vi "svx_ZScale.Multiplier Write.vi"(4 "error in (no error)":errorcluster, 5 "Value":dbl, 6 "Container State":T3, 7 "Display State In":T1={"X Scale Width %"=50.0, "Y Scale Height %"=50.0, "X-Axis Range"={"Minimum"=0.0, "Maximum"=10.0}, "Y-Axis Range"={"Minimum"=0.0, "Maximum"=10.0}, "Z-Axis Range"={"Minimum"=0.0, "Maximum"=10.0}, "Plot Color"=61212, "Frame Color"=16252785, "Background Color"=16777222, "Initial AutoScale Y"=TRUE, "AutoScale X"=2, "AutoScale Y"=2, "AutoScale Z"=2, "Plot Transparency"=FALSE, "X-Axis Name"="Frequency", "Y-Axis Name"="Amplitude", "Z-Axis Name"="", "X-Axis Scaling Factor"={"Offset"=0.0, "Multiplier"=1.0}, "Y-Axis Scaling Factor"={"Offset"=0.0, "Multiplier"=1.0}, "Z-Axis Scaling Factor"={"Offset"=0.0, "Multiplier"=1.0}, "X-Scale Visible"=TRUE, "Y-Scale Visible"=TRUE, "Z-Scale Visible"=TRUE, "X-Scale Label Visible"=TRUE, "Y-Scale Label Visible"=TRUE, "Z-Scale Label Visible"=TRUE, "X-Axis Range Scaled"={"Minimum"=0.0, "Maximum"=10.0}, "Y-Axis Range Scaled"={"Minimum"=0.0, "Maximum"=10.0}, "Z-Axis Range Scaled"={"Minimum"=0.0, "Maximum"=10.0}, "Rev Z Order"=FALSE, "X-Scale Format Str"="%#.4g", "Y-Scale Format Str"="%#.4g", "Z-Scale Format Str"="%#.4g", "Decor color"=12369084, "Scale Range Change"=refnum, "out of state queue"=refnum, "property nodes"=refnum, "Lines"=[], "Line Properties"={"Line Color"=61212, "Line Width"=61212, "Line Style"=enum."Dash", "DisplayLines"=FALSE}} {"Line Properties"."Line Width" min=1}) -> (0 "error out":errorcluster, 3 "Display State Out":T1={"X Scale Width %"=50.0, "Y Scale Height %"=50.0, "X-Axis Range"={"Minimum"=0.0, "Maximum"=10.0}, "Y-Axis Range"={"Minimum"=0.0, "Maximum"=10.0}, "Z-Axis Range"={"Minimum"=0.0, "Maximum"=10.0}, "Plot Color"=61212, "Frame Color"=16252785, "Background Color"=16777222, "Initial AutoScale Y"=TRUE, "AutoScale X"=2, "AutoScale Y"=2, "AutoScale Z"=2, "Plot Transparency"=FALSE, "X-Axis Name"="Frequency", "Y-Axis Name"="Amplitude", "Z-Axis Name"="", "X-Axis Scaling Factor"={"Offset"=0.0, "Multiplier"=1.0}, "Y-Axis Scaling Factor"={"Offset"=0.0, "Multiplier"=1.0}, "Z-Axis Scaling Factor"={"Offset"=0.0, "Multiplier"=1.0}, "X-Scale Visible"=TRUE, "Y-Scale Visible"=TRUE, "Z-Scale Visible"=TRUE, "X-Scale Label Visible"=TRUE, "Y-Scale Label Visible"=TRUE, "Z-Scale Label Visible"=TRUE, "X-Axis Range Scaled"={"Minimum"=0.0, "Maximum"=10.0}, "Y-Axis Range Scaled"={"Minimum"=0.0, "Maximum"=10.0}, "Z-Axis Range Scaled"={"Minimum"=0.0, "Maximum"=10.0}, "Rev Z Order"=FALSE, "X-Scale Format Str"="%#.4g", "Y-Scale Format Str"="%#.4g", "Z-Scale Format Str"="%#.4g", "Decor color"=12369084, "Scale Range Change"=refnum, "out of state queue"=refnum, "property nodes"=refnum, "Lines"=[], "Line Properties"={"Line Color"=61212, "Line Width"=61212, "Line Style"=enum."Dash", "DisplayLines"=FALSE}} {"Line Properties"."Line Width" min=1})   [LabVIEW 2017, in "SVX Waterfall Graph.xctl"]
uses:
  <vilib>/addons/_XControls/Waterfall Graph/SVX Waterfall Graph.xctl
  <vilib>/_xctls/Container State.ctl
  <vilib>/addons/_XControls/Waterfall Graph/subVIs/svx_Waterfall State.ctl
  <vilib>/addons/_NISVFA/_Shared subVIs/Controls/svc_Cluster of Array of Cluster of XYZ.ctl
  <vilib>/_xctls/XControlSupport.lvlib
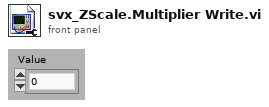
[diagram p1: front panel]
types:
  T1 = typedef "SVX Waterfall Graph.xctl/svx_Waterfall State.ctl" = cluster{"X Scale Width %":dbl, "Y Scale Height %":dbl, "X-Axis Range":cluster{"Minimum":dbl, "Maximum":dbl}, "Y-Axis Range":cluster{"Minimum":dbl, "Maximum":dbl}, "Z-Axis Range":cluster{"Minimum":dbl, "Maximum":dbl}, "Plot Color":u32, "Frame Color":u32, "Background Color":u32, "Initial AutoScale Y":bool, "AutoScale X":u8, "AutoScale Y":u8, "AutoScale Z":u8, "Plot Transparency":bool, "X-Axis Name":string, "Y-Axis Name":string, "Z-Axis Name":string, "X-Axis Scaling Factor":cluster{"Offset":dbl, "Multiplier":dbl}, "Y-Axis Scaling Factor":cluster{"Offset":dbl, "Multiplier":dbl}, "Z-Axis Scaling Factor":cluster{"Offset":dbl, "Multiplier":dbl}, "X-Scale Visible":bool, "Y-Scale Visible":bool, "Z-Scale Visible":bool, "X-Scale Label Visible":bool, "Y-Scale Label Visible":bool, "Z-Scale Label Visible":bool, "X-Axis Range Scaled":cluster{"Minimum":dbl, "Maximum":dbl}, "Y-Axis Range Scaled":cluster{"Minimum":dbl, "Maximum":dbl}, "Z-Axis Range Scaled":cluster{"Minimum":dbl, "Maximum":dbl}, "Rev Z Order":bool, "X-Scale Format Str":string, "Y-Scale Format Str":string, "Z-Scale Format Str":string, "Decor color":u32, "Scale Range Change":refnum<user-event>, "out of state queue":refnum<queue>, "property nodes":refnum<queue>, "Lines":T2[], "Line Properties":cluster{"Line Color":u32, "Line Width":u16, "Line Style":enum32{"Solid", "Dash", "Dot", "DashDot", "DashDotDot"}, "DisplayLines":bool}}
  T2 = typedef "svc_Cluster of Array of Cluster of XYZ.ctl" = cluster{"line":cluster{"X":dbl, "Y":dbl, "Z":dbl}[]}
  T3 = typedef "XControlSupport.lvlib/Container State.ctl" = cluster{"Indicator?":bool, "Run Mode?":bool, " Refnum":refnum<vi>}
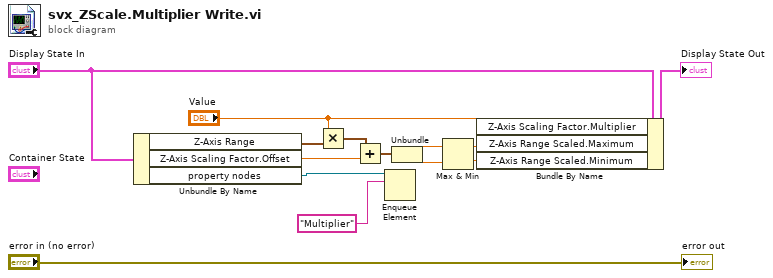
[diagram p0: block diagram]
diagram:
  n1 = Unbundle By Name("Display State In") -> ("Z-Axis Range"=w6:cluster{"Minimum":dbl, "Maximum":dbl}, "Z-Axis Scaling Factor.Offset"=w7:dbl, "property nodes"=w1:refnum<queue>)
  n2 = Multiply(x="Value", y=w6) -> (x*y=w8:cluster{"Minimum":dbl, "Maximum":dbl})
  n3 = Add(x=w8, y=w7) -> (x+y=w11:cluster{"Minimum":dbl, "Maximum":dbl})
  n4 = Enqueue Element(queue=w1, element="Multiplier" ("Property Name")) -> ()  [unwired: 2 in, 3 out]
  n5 = Unbundle(w11) -> ("Minimum"=w10:dbl, "Maximum"=w9:dbl)
  n6 = Max & Min(x=w10, y=w9) -> (max(x,y)=w12:dbl, min(x,y)=w13:dbl)
  n7 = Bundle By Name(cluster="Display State In", "Z-Axis Scaling Factor.Multiplier"="Value", "Z-Axis Range Scaled.Maximum"=w12, "Z-Axis Range Scaled.Minimum"=w13) -> (→"Display State Out":T1)
  "error out" <- "error in (no error)"
